vi "CreateActionQueues.vi"(8 "Error In":errorcluster) -> (0 "Error Out":errorcluster, 3 "Message Queues":T1)   [LabVIEW 2012]
uses:
  ActionQueues.ctl
  UIActionQueueElement.ctl
  UIAction.ctl
  HardwareActionQueueElement.ctl
  HardwareAction.ctl
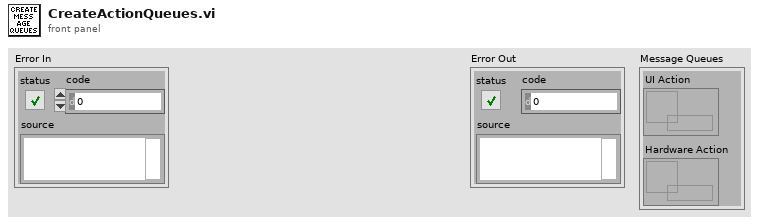
[diagram p1: front panel]
types:
  T1 = typedef "ActionQueues.ctl" = cluster{"UI Action":refnum<queue>, "Hardware Action":refnum<queue>}
  T2 = typedef "HardwareActionQueueElement.ctl" = cluster{"State":T3, "Data":variant}
  T3 = typedef "HardwareAction.ctl" = enum16{"Initialize", "Start", "Read", "Write", "Stop", "Shutdown"}
  T4 = typedef "UIActionQueueElement.ctl" = cluster{"Action":T5, "Data":variant}
  T5 = typedef "UIAction.ctl" = enum16{"Initialize", "Connected", "Select Pattern", "Update Patterns", "Error", "Shutdown"}
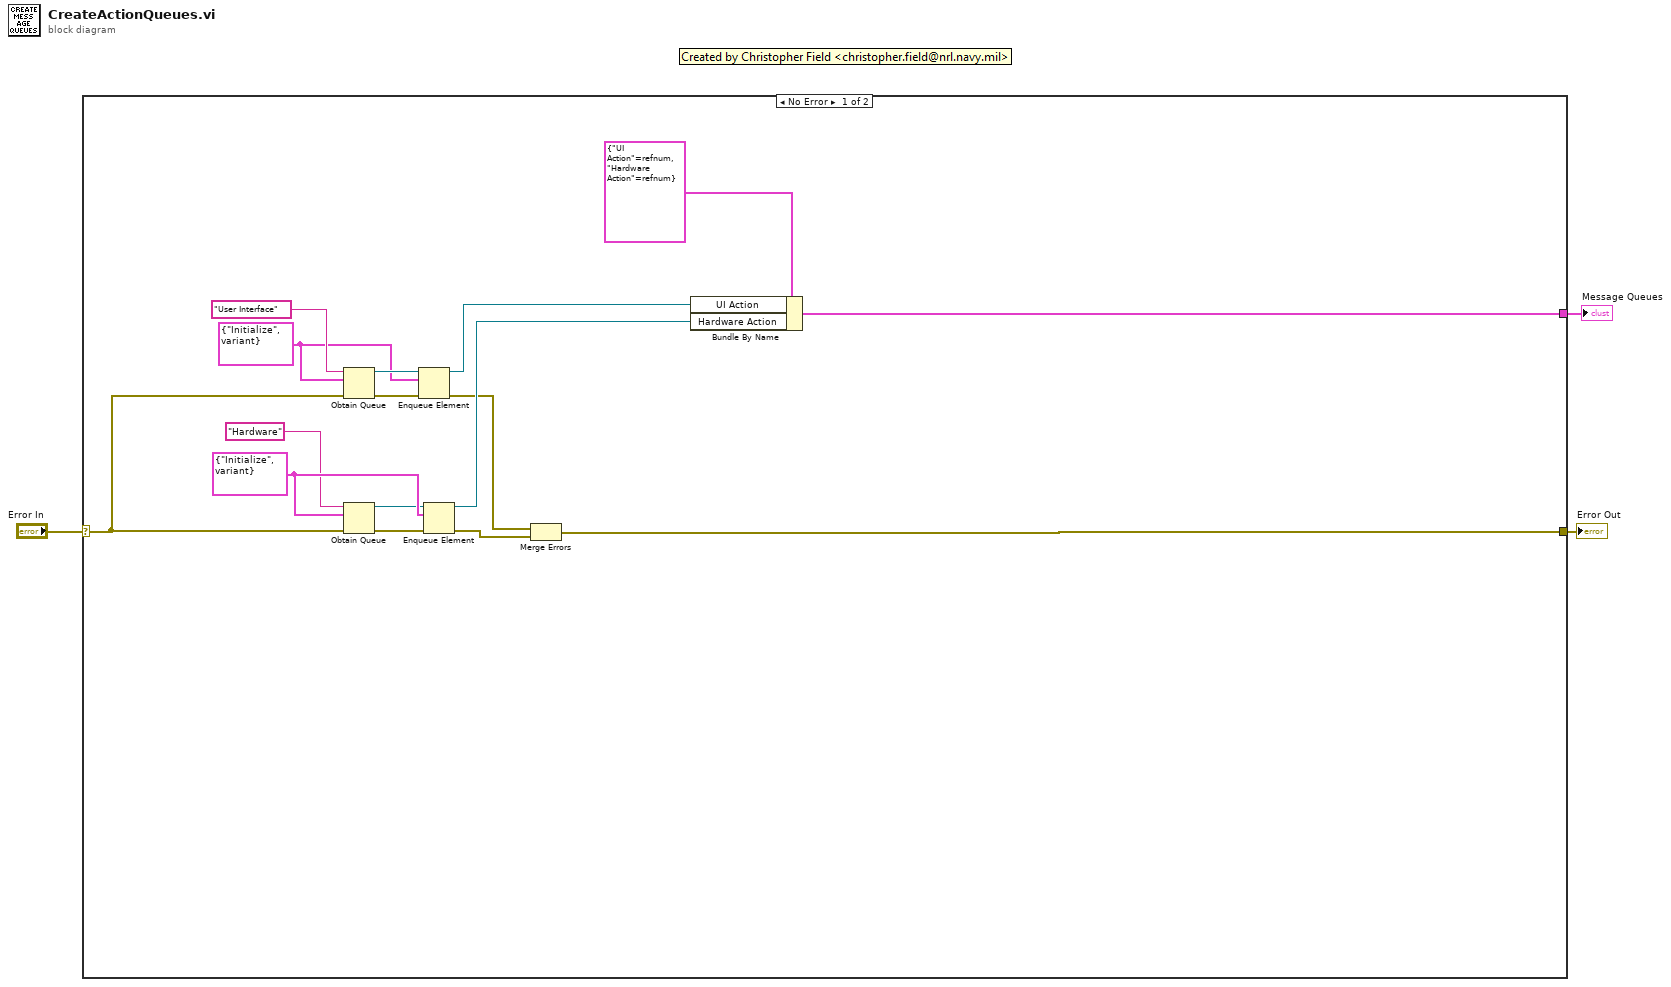
[diagram p0: block diagram]
diagram:
  n1 = case shown="No Error" "Error In" {
    selector: "Error In" -> [w13 w20]
    tunnel: [w5 w20] -> w2
    tunnel: [w4 _] -> w1
    frame No Error {
      w15 = T2 {"State"=enum."Initialize", "Data"=variant} ("Acquisition Queue Element")
      w16 = T4 {"Action"=enum."Initialize", "Data"=variant} ("User Interface Queue Element")
      n2 = Obtain Queue(name (unnamed)="User Interface", element data type=w16, error in (no error)=w13) -> (queue out=w18:refnum<queue>, error out=w17:errorcluster)  [unwired: 2 in, 1 out]
      n3 = Obtain Queue(name (unnamed)="Hardware", element data type=w15, error in (no error)=w13) -> (queue out=w14:refnum<queue>, error out=w12:errorcluster)  [unwired: 2 in, 1 out]
      n4 = Enqueue Element(queue=w18, element=w16, error in (no error)=w17) -> (queue out=w9:refnum<queue>, error out=w7:errorcluster)  [unwired: 1 in, 1 out]
      n5 = Enqueue Element(queue=w14, element=w15, error in (no error)=w12) -> (queue out=w8:refnum<queue>, error out=w6:errorcluster)  [unwired: 1 in, 1 out]
      n6 = Merge Errors(w7, w6) -> (w5:errorcluster)
      n7 = Bundle By Name(cluster=T1 {"UI Action"=refnum, "Hardware Action"=refnum} ("Message Queues"), "UI Action"=w9, "Hardware Action"=w8) -> (w4:T1)
    }
    frame Error {
    }
  }
  "Error Out" <- w2
  "Message Queues" <- w1
